vi "Configure Time Domain Trace Coupling.vi"(8 "error in (no error)":errorcluster, 9 "Enable Time Domain Trace Coupling (T: Enable)":bool=TRUE, 10 "Channel (1)":i32=1, 11 "VISA resource name":refnum<visa-resource-name>) -> (0 "error out":errorcluster, 3 "VISA resource name out":refnum<visa-resource-name>)   [LabVIEW 2018, in "Keysight PNA Series.lvlib"]
doc: "Configures Time Domain Trace Coupling."
uses:
  Keysight PNA Series.lvlib
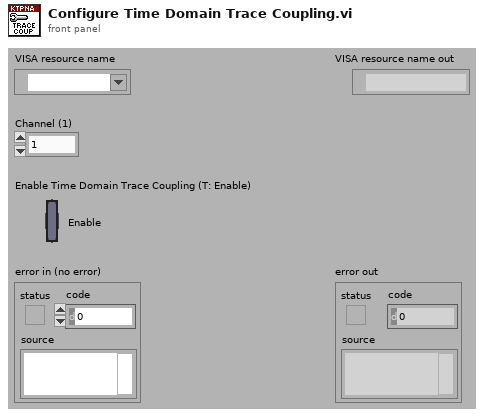
[diagram p1: front panel]
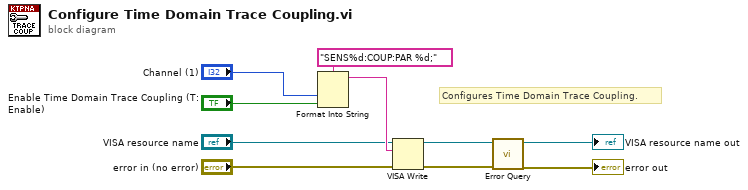
[diagram p0: block diagram]
diagram:
  # "Configures Time Domain Trace Coupling."
  n1 = Format Into String(format string="SENS%d:COUP:PAR %d;", "Channel (1)", "Enable Time Domain Trace Coupling (T: Enable)") -> (resulting string=w8:string)  [unwired: 2 in, 1 out]
  n2 = VISA Write(VISA resource name="VISA resource name", write buffer=w8, error in (no error)="error in (no error)") -> (VISA resource name out=w5:refnum<visa-resource-name>, error out=w4:errorcluster)  [unwired: 1 out]
  n3 = call "Error Query.vi"("error in (no error)"=w4, "VISA resource name"=w5) -> ("error out"=→"error out":errorcluster, "VISA resource name out"=→"VISA resource name out":refnum<visa-resource-name>)  [unwired: 6 in, 2 out]
